vi "Turn.vi"(6 "Error":errorcluster, 7 "Actor":refnum<class "Actor.lvclass">, 10 "MsgDVR":refnum<data-value>, 11 "Actor":T1) -> (3 "Actor":T1, 4 "Error":errorcluster, 5 "Actor":refnum<class "Actor.lvclass">)   [LabVIEW 2020, in "jettl.lvlib"]
uses:
  jettl.lvlib
  Actor/Actor.lvclass
  Msg.ctl
  Msg/Msg.lvclass
  Origin.ctl
  Metadata/Metadata.lvclass
  Lifecycle.ctl
  MsgAttribs.ctl
  MsgExecuteType.ctl
  PostSetup.ctl
  PreSetup.ctl
  MsgNames.ctl
  ActorAttribs.ctl
  ChildActors.ctl
  Actor.ctl
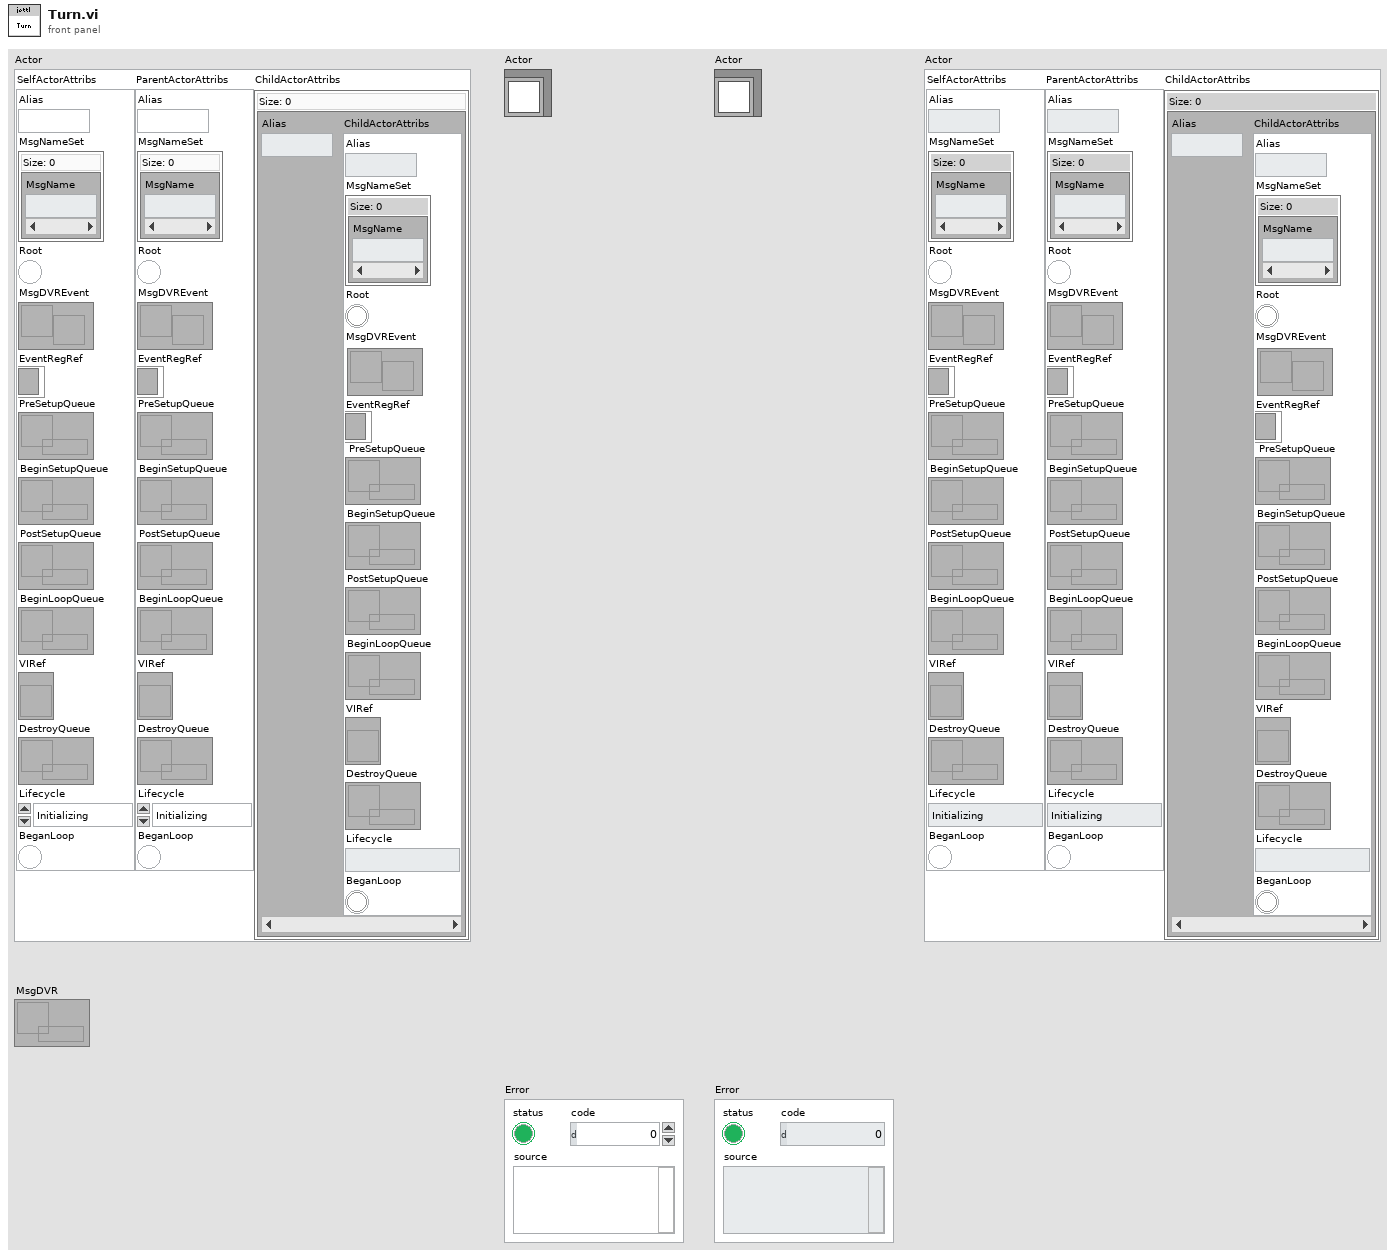
[diagram p1: front panel]
types:
  T1 = typedef "jettl.lvlib/Actor.ctl" = cluster{"SelfActorAttribs":T2, "ParentActorAttribs":T2, "ChildActorAttribs":T5}
  T2 = typedef "jettl.lvlib/ActorAttribs.ctl" = cluster{"Alias":string, "MsgNameSet":T3, "Root":bool, "MsgDVREvent":refnum<user-event>, "EventRegRef":refnum<event-registration>, "PreSetupQueue":refnum<queue>, "BeginSetupQueue":refnum<queue>, "PostSetupQueue":refnum<queue>, "BeginLoopQueue":refnum<queue>, "VIRef":refnum<vi>, "DestroyQueue":refnum<queue>, "Lifecycle":T4, "BeganLoop":bool}
  T3 = typedef "jettl.lvlib/MsgNames.ctl" = set{string}
  T4 = typedef "jettl.lvlib/Lifecycle.ctl" = enum16{"Initializing", "SettingUp", "Starting", "Running", "Stopping", "TearingDown", "Terminated"}
  T5 = typedef "jettl.lvlib/ChildActors.ctl" = map{string, T2}
  T6 = typedef "jettl.lvlib/Msg.ctl" = cluster{"MsgAttribsDVR":refnum<data-value>, "Msg":refnum<class "Msg.lvclass">}
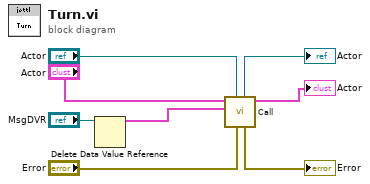
[diagram p0: block diagram]
diagram:
  n1 = Delete Data Value Reference(data value reference="MsgDVR") -> (data value=w5:T6)  [unwired: 1 in, 1 out]
  n2 = call "Call.vi"("Error"="Error", 7:"Actor"="Actor", "Msg"=w5, 11:"Actor"="Actor") -> (3:"Actor"=→"Actor":T1, "Error"=→"Error":errorcluster, 5:"Actor"=→"Actor":refnum<class "Actor.lvclass">)  [unwired: 5 in]
